vi "MC5e Open Squad XML.vi"(8 "error in":errorcluster, 9 "Cancelled?":bool, 11 "selected path":path) -> (0 "error out":errorcluster, 3 "Squad Array":T1[](array[typedef]) {"CR" items=["30", "29", "28", "27", "26", "25", "24", "23", "22", "21", "20", "19", "18", "17", "16", "15", "14", "13", "12", "11", "10", "9", "8", "7", "6", "5", "4", "3", "2", "1", "1/2", "1/4", "1/8"]})   [LabVIEW 2020]
uses:
  MC5e Squad_Info.ctl
  MC5e Size_Categories.ctl
  MC5e Global_Error_Codes.vi
panel:
  # "Squads are restricted to one type of soldier (i.e  Archers) and all of the same level.\nIf you want mixed CR or mixed types, use multiple squads."
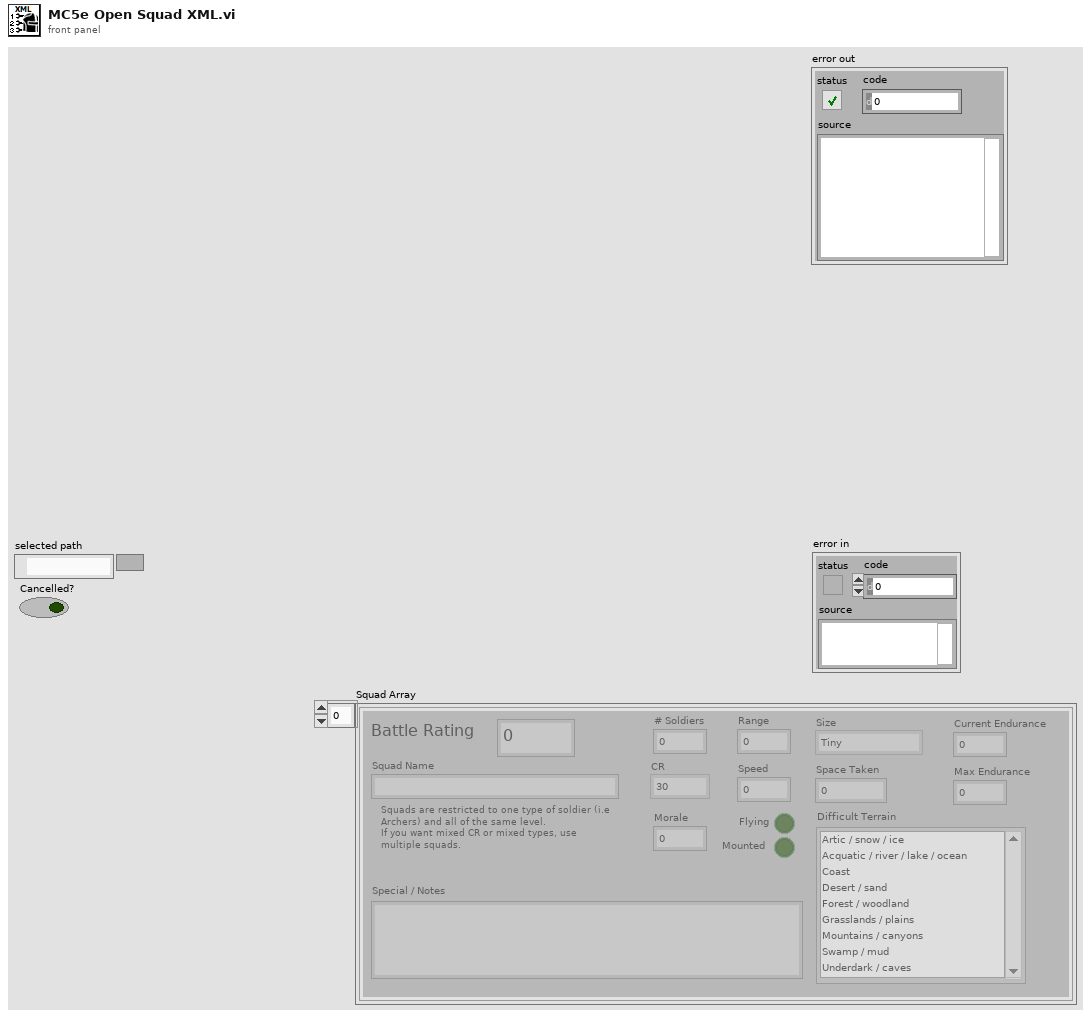
[diagram p1: front panel]
types:
  T1 = typedef "MC5e Squad_Info.ctl" = cluster{"Squad Name":string, "# Soldiers":u16, "Battle Rating":u16, "Flying":bool, "Mounted":bool, "Speed":u16, "Range":u16, "Morale":i32, "Max Endurance":u16, "Current Endurance":i32, "Size":T2, "Space Taken":u16, "Difficult Terrain":i32[], "CR":u16, "Special / Notes":string}
  T2 = typedef "MC5e Size_Categories.ctl" = enum16{"Tiny", "Small", "Medium", "Large", "Huge", "Gargantuan"}
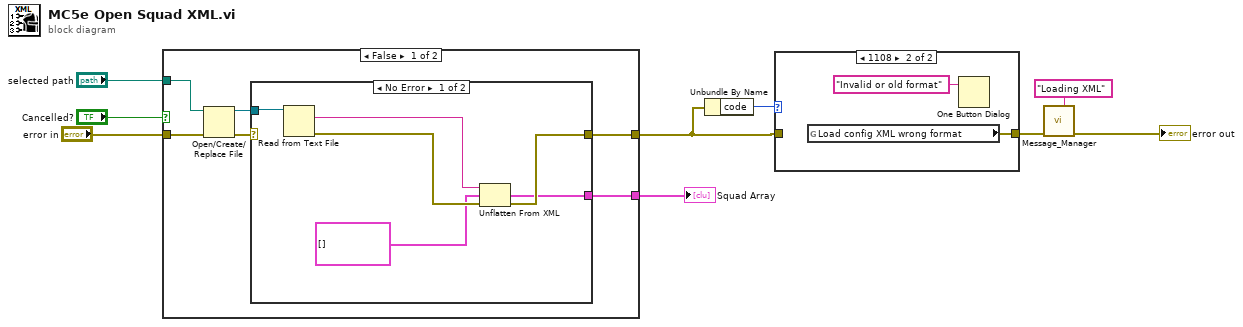
[diagram p0: block diagram]
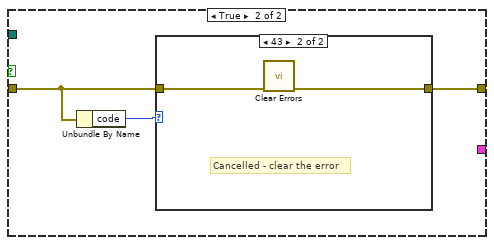
[diagram p4: hidden frame]
diagram:
  n1 = case shown="False" "Cancelled?" {
    tunnel: [w15 w23] -> w8
    tunnel: "selected path" -> [w14 _]
    tunnel: "error in" -> [w10 w24]
    tunnel: [w11 _] -> w7
    frame False {
      n2 = Open/Create/Replace File(file path (use dialog)=w14, error in=w10) -> (refnum out=w12:refnum<file>, error out=w13:errorcluster)  [unwired: 4 in, 1 out]
      n3 = case shown="No Error" w13 {
        selector: w13 -> [_ w22]
        tunnel: [w21 w22] -> w15
        tunnel: w12 -> [w20 _]
        tunnel: [w17 _] -> w11
        frame No Error {
          n4 = Read from Text File(file (use dialog)=w20) -> (text=w19:string, error out=w18:errorcluster)  [unwired: 3 in, 2 out]
          n5 = Unflatten From XML(xml string=w19, type=T1[] [], error in (no error)=w18) -> (value=w17:T1[], error out=w21:errorcluster)
        }
        frame Error {
        }
      }
    }
    frame True {
      n6 = Unbundle By Name(w24) -> ("code"=w25:i32)
      n7 = case shown="43" w25 {
        tunnel: w24 -> [w26 w28]
        tunnel: [w26 w27] -> w23
        frame 0, Default {
        }
        frame 43 {
          # "Cancelled - clear the error"
          n8 = call <vilib>:"Clear Errors.vi"("error in (no error)"=w28) -> ("error out"=w27:errorcluster)  [unwired: 5 in, 1 out]
        }
      }
    }
  }
  "Squad Array" <- w7
  n9 = Unbundle By Name(w8) -> ("code"=w9:i32)
  n10 = case shown="1108" w9 {
    tunnel: [w29 w31] -> w6
    tunnel: w8 -> [w29 _]
    frame 0, Default {
    }
    frame 1108 {
      n11 = global read "MC5e Global_Error_Codes.vi" "Load config XML wrong format"() -> (w31:errorcluster)
      n12 = One Button Dialog(message="Invalid or old format") -> ()  [unwired: 1 in, 1 out]
    }
  }
  n13 = call "Message_Manager.vi"("error in"=w6, "New Entry"="Loading XML") -> ("error out"=→"error out":errorcluster)  [unwired: 5 in, 4 out]
